vi "Destroy.vi"(11 "Panel in":refnum<class "Helper Loop.lvclass">) -> (0 "error out":errorcluster)   [LabVIEW 2021, in "Helper Loop.lvclass"]
uses:
  Helper Loop.lvclass
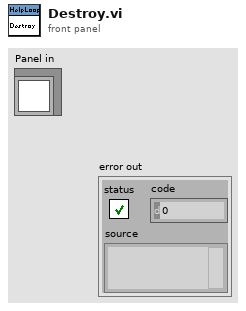
[diagram p1: front panel]
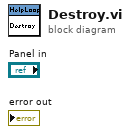
[diagram p0: block diagram]
diagram:
